vi "CreateWO-GenerateWorkOrder.vi"(0 "Work Orders":string[][](array[string])) -> (1 "Created Work Order":string)   [LabVIEW 2013, in "ERP-CreateWorkOrder.lvclass"]
uses:
  ERP-CreateWorkOrder.lvclass
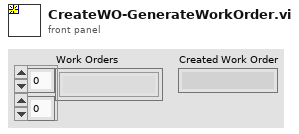
[diagram p1: front panel]
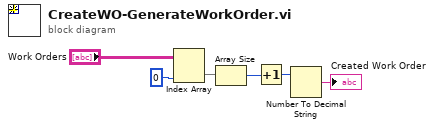
[diagram p0: block diagram]
diagram:
  n1 = Index Array(array="Work Orders", index (col)=0 ("disabled index (col)")) -> (element=w4:string[])  [unwired: 1 in]
  n2 = Array Size(array=w4) -> (size(s)=w5:i32)
  n3 = Increment(x=w5) -> (x+1=w6:i32)
  n4 = Number To Decimal String(number=w6) -> (decimal integer string=→"Created Work Order":string)  [unwired: 1 in]
